vi "ReadTCPPackage.vi"(0 "connection ID":refnum<k5>, 3 "timeout ms (200)":i32=200, 5 "error in (no error)":errorcluster) -> (15 "payload":string, 16 "command":T1 items=["GarbageCollect", "GetAllObjects", "GetAllObjectsReply", "CleanUp", "G#Event", "RegisterClient", "GetAttributeValue", "GetAttributeValueReply", "GetClassAttributeValue", "GetClassAttributeValueReply", "GetToStringValue", "GetToStringValueReply", "GetClassHierarchy", "GetClassHierarchyReply", "Destroy", "RemoveClient"], 18 "timeout":bool, 19 "error out":errorcluster)   [LabVIEW 2017, in "G#DebugServer.lvclass"]
doc: "Reads an UDP package."
uses:
  <vilib>/addons/_AddQ/G#DebugServer/G#DebugServer.lvclass
  <vilib>/addons/_AddQ/G#DebugServer/utils/TCPCommand.ctl
  <vilib>/addons/_AddQ/G#Object/G#Object.lvclass
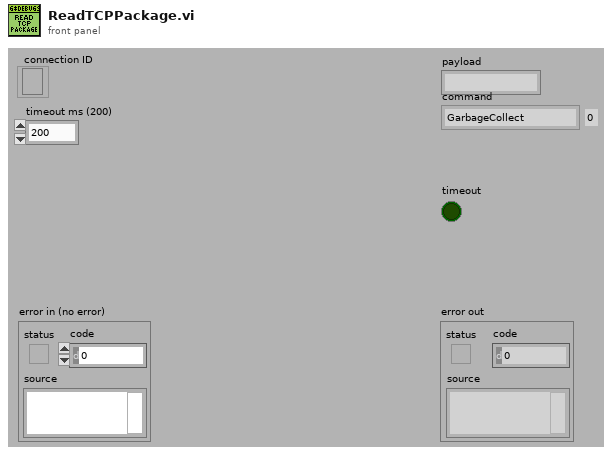
[diagram p1: front panel]
types:
  T1 = typedef "G#DebugServer.lvclass/TCPCommand.ctl" = u8
  T2 = enum16{"Standard", "Buffered", "CRLF", "Immediate"}
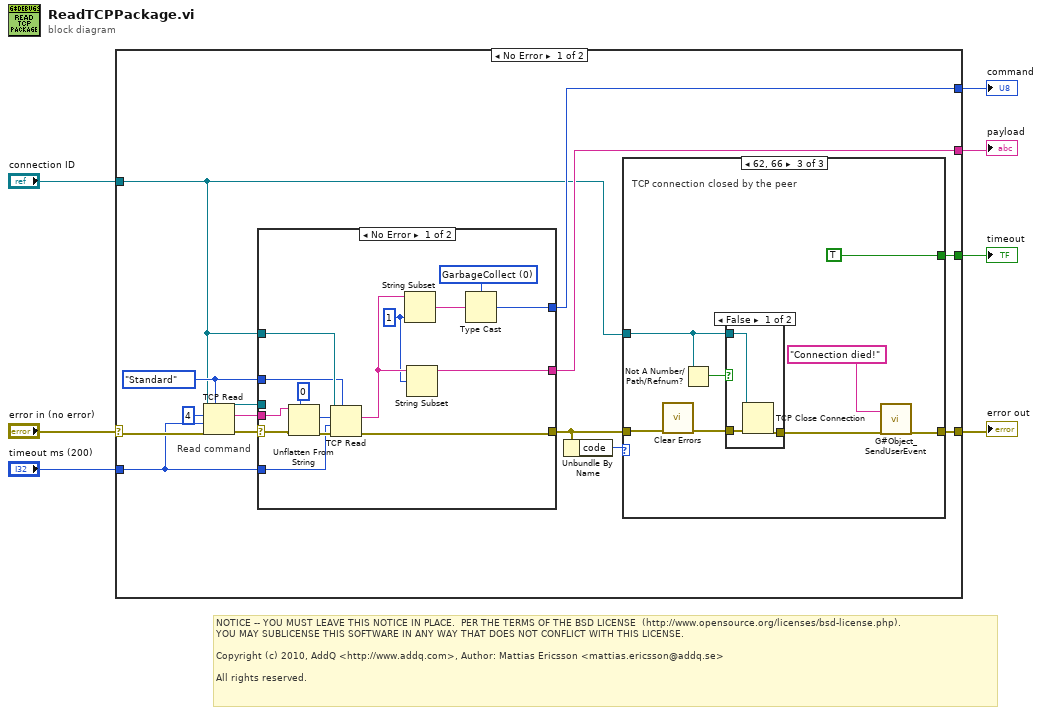
[diagram p0: block diagram]
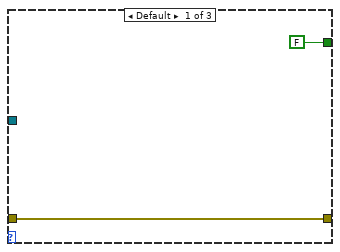
[diagram p2: hidden frame]
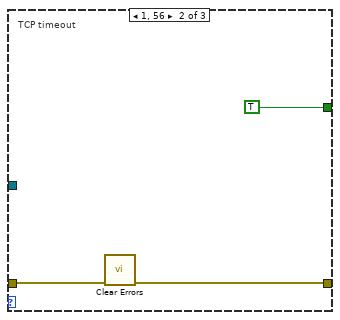
[diagram p3: hidden frame]
diagram:
  # "NOTICE -- YOU MUST LEAVE THIS NOTICE IN PLACE.  PER THE TERMS OF THE BSD LICENSE  (http://www.opensource.org/licenses/bsd-license.php).\nYOU MAY SUBLICENSE THIS SOFTWARE IN ANY WAY THAT DOES NOT CONFLICT WITH THIS LICENSE.\n\nCopyright (c) 2010, AddQ <http://www.addq.com>, Author: Mattias Ericsson <mattias.ericsson@addq.se>\n\nAll rights reserved."
  n1 = case shown="No Error" "error in (no error)" {
    selector: "error in (no error)" -> [w21 w55]
    tunnel: [w12 w55] -> w6
    tunnel: "connection ID" -> [w8 _]
    tunnel: [w20 _] -> w4
    tunnel: [w11 _] -> w3
    tunnel: [w16 _] -> w2
    tunnel: "timeout ms (200)" -> [w14 _]
    frame No Error {
      w13 = T2."Standard" ("mode (standard)")
      # "Read command"
      n2 = TCP Read(connection ID=w8, bytes to read=4, error in (no error)=w21, 7:w13, 9:w14) -> (connection ID out=w17:refnum<k5>, data out=w18:string, error out=w19:errorcluster)
      n3 = case shown="No Error" w19 {
        selector: w19 -> [w49 w54]
        tunnel: [w42 w54] -> w10
        tunnel: w18 -> [w48 _]
        tunnel: w17 -> [_ _]
        tunnel: [w52 _] -> w16
        tunnel: [w53 _] -> w20
        tunnel: w8 -> [w44 _]
        tunnel: w14 -> [w43 _]
        tunnel: w13 -> [w40 _]
        frame No Error {
          w39 = 1 ("length (rest)")
          w51 = T1 0 items=["GarbageCollect"] ("Command")
          n4 = Unflatten From String(type=0, binary string=w48, error in (no error)=w49) -> (value=w45:i32, error out=w46:errorcluster)  [unwired: 2 in, 1 out]
          n5 = TCP Read(connection ID=w44, bytes to read=w45, error in (no error)=w46, 7:w40, 9:w43) -> (data out=w41:string, error out=w42:errorcluster)  [unwired: 1 out]
          n6 = String Subset(string=w41, length (rest)=w39) -> (substring=w50:string)  [unwired: 1 in]
          n7 = String Subset(string=w41, offset (0)=w39) -> (substring=w52:string)  [unwired: 1 in]
          n8 = Type Cast(type=w51, x=w50) -> (*(type *) &x=w53:T1)
        }
        frame Error {
        }
      }
      n9 = Unbundle By Name(w10) -> ("code"=w9:i32)
      n10 = case shown="62, 66" w9 {
        tunnel: w10 -> [w22 w26 w34]
        tunnel: [w22 w25 w31] -> w12
        tunnel: [FALSE TRUE TRUE] -> w11
        tunnel: w8 -> [_ _ w28]
        frame Default {
        }
        frame 1, 56 {
          # "TCP timeout"
          n11 = call <vilib>:"Clear Errors.vi"("error in (no error)"=w26) -> ("error out"=w25:errorcluster)  [unwired: 5 in, 1 out]
        }
        frame 62, 66 {
          # "TCP connection closed by the peer"
          n12 = call <vilib>:"Clear Errors.vi"("error in (no error)"=w34) -> ("error out"=w32:errorcluster)  [unwired: 5 in, 1 out]
          n13 = Not A Number/Path/Refnum?(number/path/refnum=w28) -> (NaN/Path/Refnum?=w27:bool)
          n14 = case shown="False" w27 {
            tunnel: w32 -> [w37 w38]
            tunnel: [w36 w38] -> w30
            tunnel: w28 -> [w35 _]
            frame False {
              n15 = TCP Close Connection(connection ID=w35, error in (no error)=w37) -> (error out=w36:errorcluster)  [unwired: 1 in, 1 out]
            }
            frame True {
            }
          }
          n16 = call <vilib>:"G#Object_SendUserEvent.vi"("text"="Connection died!", "error in (no error)"=w30) -> ("error out"=w31:errorcluster)  [unwired: 16 in, 1 out]
        }
      }
    }
    frame Error {
    }
  }
  "error out" <- w6
  "payload" <- w2
  "command" <- w4
  "timeout" <- w3
